vi "DefectArrays.vi"(0 "action":enum16{"Nothing", "Write", "Read", "Initialise"}(ring), 1 "Region Index":i32, 2 "Defect array IN":i32[][](graph)) -> (3 "Defect array OUT":i32[][](graph), 4 "Region Indices":i32[](array[numeric]), 5 "To":i32[](array[numeric]), 6 "Maximum":i32, 7 "max. No. of points in region":i32, 8 "From":i32[](array[numeric]), 9 "No. of points in region":i32[](array[numeric]), 10 "Minimum":i32)   [LabVIEW 2018]
uses:
  ProbePlan/ProbePlanParams.vi
panel:
  out "Array - Numeric":i32[][](array[numeric])
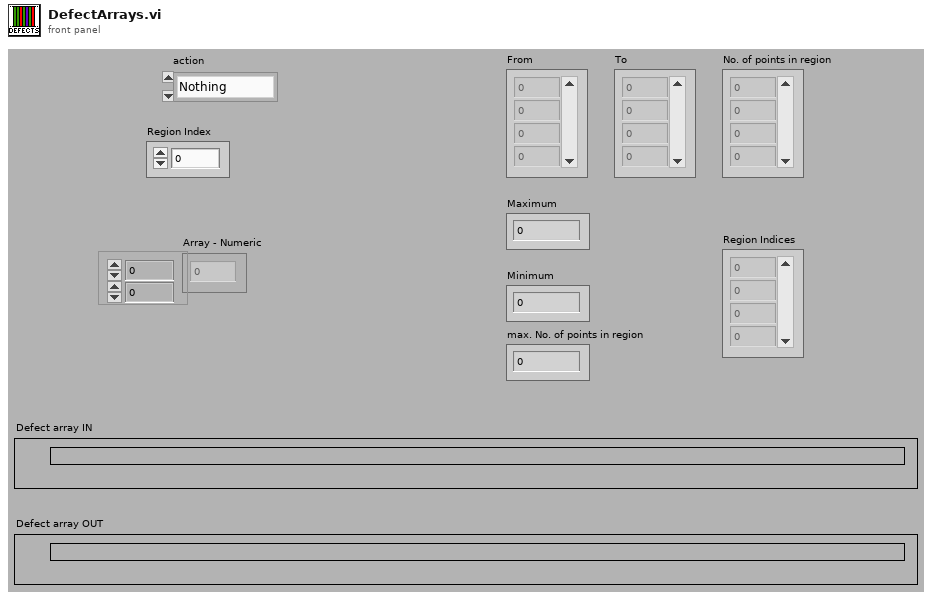
[diagram p1: front panel]
types:
  T1 = cluster{"Strip Number OUT":i32, "X0":i32, "Y0":i32, "X1":i32, "Y1":i32, "Xref":dbl, "Yref":dbl, "ProbePlan type":u32, "Inner pads offset":ext, "Outer pads offset":ext, "l_inner":ext, "l_outer":ext, "strip numbering":u16, "Device Orientation":ext, "Stagger offset":i32, "Yoffset":dbl, "Strip pitch":dbl, "Fiducail separation":dbl, "Radius":ext, "Relative strip angles":dbl, "Probeplan description":string, "ProbePlan array":cluster{"Region":string, "ProbePoints":cluster{"X":dbl, "Y":dbl, "Label":string, "CardViable?":bool}[]}[], "Test ProbePoints":cluster{"Regions Enabled":bool[], "From index":u32[], "To index":u32[], "Strip length [cm]":dbl[]}}
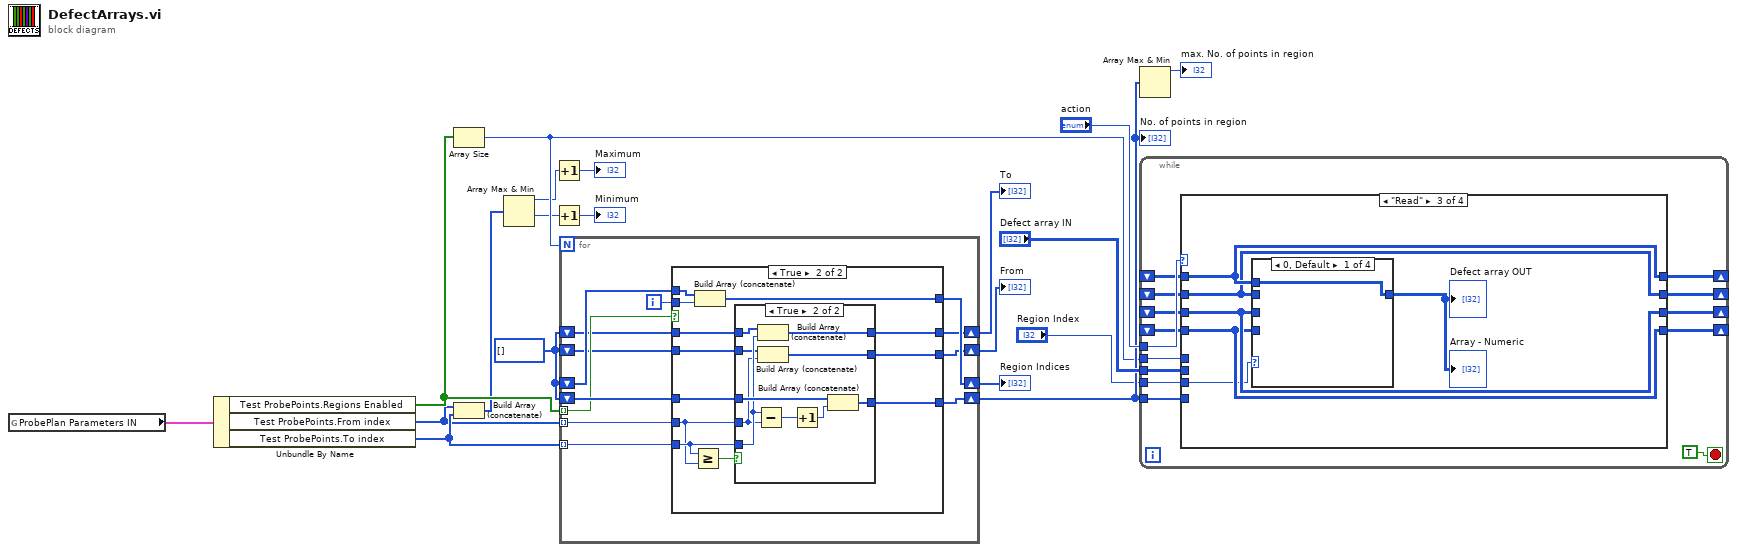
[diagram p0: block diagram]
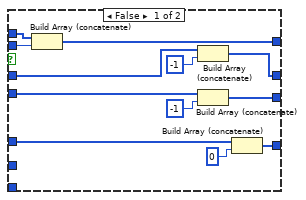
[diagram p2: hidden frame]
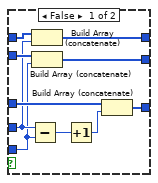
[diagram p3: hidden frame]
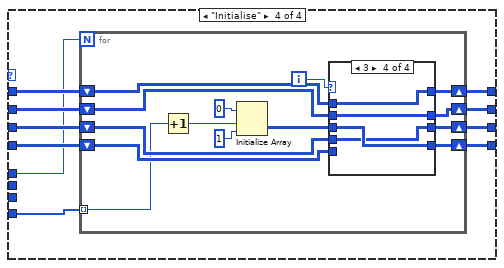
[diagram p12: hidden frame]
diagram:
  w9 = i32[] []
  n1 = global read "ProbePlanParams.vi" "ProbePlan Parameters IN"() -> (w17:T1)
  n2 = Unbundle By Name(w17) -> ("Test ProbePoints.Regions Enabled"=w16:bool[], "Test ProbePoints.From index"=w13:u32[], "Test ProbePoints.To index"=w14:u32[])
  n3 = Array Size(array=w16) -> (size(s)=w5:i32)
  n4 = Build Array (concatenate)(w13, w14) -> (w12:u32[])
  n5 = Array Max & Min(array=w12) -> (max value=w4:u32, min value=w2:u32)  [unwired: 2 out]
  n6 = Increment(x=w4) -> (x+1=→"Maximum":u32)
  n7 = Increment(x=w2) -> (x+1=→"Minimum":u32)
  n8 = for {
    N: w5 -> [_]
    tunnel: w16 -> [w27] mode=indexing
    tunnel: w13 -> [w28] mode=indexing
    tunnel: w14 -> [w29] mode=indexing
    shift-right: [w30] -> w11
    shift-left: w9 -> [w31]
    shift-right: [w24] -> w10
    shift-left: w9 -> [w25]
    shift-right: [w20] -> w7
    shift-left: w9 -> [w23]
    shift-right: [w21] -> w8
    shift-left: w9 -> [w22]
    i -> [w26]
    n9 = case shown="True" w27 {
      tunnel: w31 -> [w37 w55]
      tunnel: [w35 w53] -> w30
      tunnel: w29 -> [_ w52]
      tunnel: w28 -> [_ w51]
      tunnel: w26 -> [w34 w49]
      tunnel: w25 -> [w33 w50]
      tunnel: [w32 w48] -> w24
      tunnel: w23 -> [w42 w47]
      tunnel: w22 -> [w43 w46]
      tunnel: [w39 w45] -> w21
      tunnel: [w38 w44] -> w20
      frame False {
        n10 = Build Array (concatenate)(w33, w34) -> (w32:i32[])
        n11 = Build Array (concatenate)(w43, -1) -> (w39:u32[])
        n12 = Build Array (concatenate)(w42, -1) -> (w38:u32[])
        n13 = Build Array (concatenate)(w37, 0) -> (w35:u32[])
      }
      frame True {
        n14 = Greater Or Equal?(x=w52, y=w51) -> (x >= y?=w54:bool)
        n15 = Build Array (concatenate)(w50, w49) -> (w48:i32[])
        n16 = case shown="True" w54 {
          tunnel: w55 -> [w64 w75]
          tunnel: [w62 w72] -> w53
          tunnel: w52 -> [w56 w71]
          tunnel: w51 -> [w60 w70]
          tunnel: w47 -> [w61 w69]
          tunnel: w46 -> [w59 w68]
          tunnel: [w58 w67] -> w45
          tunnel: [w57 w66] -> w44
          frame False {
            n17 = Subtract(x=w60, y=w56) -> (x-y=w65:u32)
            n18 = Build Array (concatenate)(w59, w60) -> (w58:u32[])
            n19 = Build Array (concatenate)(w61, w56) -> (w57:u32[])
            n20 = Increment(x=w65) -> (x+1=w63:u32)
            n21 = Build Array (concatenate)(w64, w63) -> (w62:u32[])
          }
          frame True {
            n22 = Subtract(x=w71, y=w70) -> (x-y=w74:u32)
            n23 = Build Array (concatenate)(w68, w71) -> (w67:u32[])
            n24 = Build Array (concatenate)(w69, w70) -> (w66:u32[])
            n25 = Increment(x=w74) -> (x+1=w73:u32)
            n26 = Build Array (concatenate)(w75, w73) -> (w72:u32[])
          }
        }
      }
    }
  }
  "From" <- w7
  "To" <- w8
  "No. of points in region" <- w11
  "Region Indices" <- w10
  n27 = Array Max & Min(array=w11) -> (max value=→"max. No. of points in region":u32)  [unwired: 3 out]
  n28 = while {
    shift-right: [w88] -> _
    shift-left: _ -> [w84]
    shift-right: [w87] -> _
    shift-left: _ -> [w83]
    shift-right: [w86] -> _
    shift-left: _ -> [w82]
    shift-right: [w85] -> _
    shift-left: _ -> [w81]
    tunnel: "action" -> [w89]
    tunnel: "Defect array IN" -> [w80]
    tunnel: w11 -> [w77]
    tunnel: "Region Index" -> [w78]
    tunnel: w5 -> [w76]
    stop <- TRUE stop-if-true
    n29 = case shown="\"Read\"" w89 {
      tunnel: [w93 w102 w125 w139] -> w88
      tunnel: [w92 w101 w124 w138] -> w87
      tunnel: [w91 w100 w123 w137] -> w86
      tunnel: [w90 w99 w122 w136] -> w85
      tunnel: w84 -> [w93 w95 w125 w135]
      tunnel: w83 -> [w92 w98 w124 w134]
      tunnel: w82 -> [w91 w97 w123 w133]
      tunnel: w81 -> [w90 w96 w122 w132]
      tunnel: w80 -> [_ w103 _ _]
      tunnel: w78 -> [_ w94 w121 _]
      tunnel: w77 -> [_ _ _ w130]
      tunnel: w76 -> [_ _ _ w131]
      frame "Nothing", Default {
      }
      frame "Write" {
        n30 = case shown="3" w94 {
          tunnel: w103 -> [w107 w111 w115 w119]
          tunnel: [w107 w110 w114 w118] -> w102
          tunnel: [w106 w111 w113 w117] -> w101
          tunnel: [w105 w109 w115 w116] -> w100
          tunnel: [w104 w108 w112 w119] -> w99
          tunnel: w98 -> [w106 _ w113 w117]
          tunnel: w97 -> [w105 w109 _ w116]
          tunnel: w96 -> [w104 w108 w112 _]
          tunnel: w95 -> [_ w110 w114 w118]
          frame 0, Default {
          }
          frame 1 {
          }
          frame 2 {
          }
          frame 3 {
          }
        }
      }
      frame "Read" {
        n31 = case shown="0, Default" w121 {
          tunnel: w125 -> [w126 _ _ _]
          tunnel: [w126 w127 w128 w129] -> w120
          tunnel: w124 -> [_ w127 _ _]
          tunnel: w123 -> [_ _ w128 _]
          tunnel: w122 -> [_ _ _ w129]
          frame 0, Default {
          }
          frame 1 {
          }
          frame 2 {
          }
          frame 3 {
          }
        }
        "Defect array OUT" <- w120
        "Array - Numeric" <- w120
      }
      frame "Initialise" {
        n32 = for {
          N: w131 -> [_]
          tunnel: w130 -> [w141] mode=indexing
          shift-right: [w151] -> w139
          shift-left: w135 -> [w147]
          shift-right: [w150] -> w138
          shift-left: w134 -> [w146]
          shift-right: [w149] -> w137
          shift-left: w133 -> [w145]
          shift-right: [w148] -> w136
          shift-left: w132 -> [w144]
          i -> [w142]
          n33 = Increment(x=w141) -> (x+1=w140:u32)
          n34 = Initialize Array(0, w140, 1) -> (w152:i32[][])
          n35 = case shown="3" w142 {
            tunnel: w152 -> [w157 w161 w165 w169]
            tunnel: [w157 w160 w164 w168] -> w151
            tunnel: [w156 w161 w163 w167] -> w150
            tunnel: [w155 w159 w165 w166] -> w149
            tunnel: [w154 w158 w162 w169] -> w148
            tunnel: w147 -> [_ w160 w164 w168]
            tunnel: w146 -> [w156 _ w163 w167]
            tunnel: w145 -> [w155 w159 _ w166]
            tunnel: w144 -> [w154 w158 w162 _]
            frame 0, Default {
            }
            frame 1 {
            }
            frame 2 {
            }
            frame 3 {
            }
          }
        }
      }
    }
  }
